vi "SMSMagnet.ProcEvents.vi"(0 "i ref in":refnum<vi>, 5 "error in (no error)":errorcluster) -> (14 "i ref out":refnum<vi>, 19 "error out":errorcluster)   [LabVIEW 2014, in "SMSMagnet.lvlib"]
doc: "This method is used to define the events the object will listen to. Add your own events here."
uses:
  SMSMagnet.lvlib
  CSCore/BaseProcess/BaseProcess.event definition.ctl
  CSCore/CAEObj/CAEObj.event definition.ctl
  CSCore/BaseProcess/BaseProcess.descriptor string definition.ctl
  CSCore/BaseProcess/BaseProcess.lvlib
  CSCore/CAEObj/CAEObj.lvlib
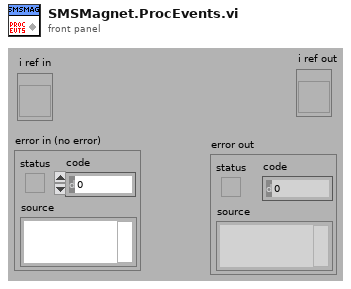
[diagram p1: front panel]
types:
  T1 = typedef "BaseProcess.lvlib/BaseProcess.event definition.ctl" = cluster{"CAEEvtDef":T2, "Data Descriptor":T3}
  T2 = typedef "CAEObj.lvlib/CAEObj.event definition.ctl" = cluster{"URL":string, "enable":bool, "ignoreResID":bool}
  T3 = typedef "BaseProcess.lvlib/BaseProcess.descriptor string definition.ctl" = string
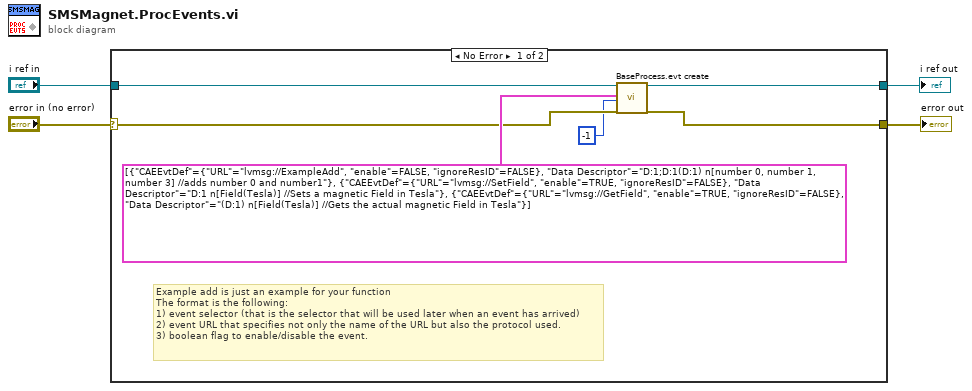
[diagram p0: block diagram]
diagram:
  n1 = case shown="No Error" "error in (no error)" {
    selector: "error in (no error)" -> [w6 w11]
    tunnel: "i ref in" -> [w10 w12]
    tunnel: [w9 w12] -> w3
    tunnel: [w8 w11] -> w2
    frame No Error {
      # "Example add is just an example for your function\nThe format is the following:\n1) event selector (that is the selector that will be used later when an event has arrived)\n2) event URL that specifies not only the name of the URL but also the protocol used.\n3) boolean flag to enable/disable the event."
      n2 = call "BaseProcess.evt create.vi"("i ref in"=w10, "newEvents"=T1[] [{"CAEEvtDef"={"URL"="lvmsg://ExampleAdd", "enable"=FALSE, "ignoreResID"=FALSE}, "Data Descriptor"="D:1;D:1(D:1) n[number 0, number 1, number 3] //adds number 0 and number1"}, {"CAEEvtDef"={"URL"="lvmsg://SetField", "enable"=TRUE, "ignoreResID"=FALSE}, "Data Descriptor"="D:1 n[Field(Tesla)] //Sets a magnetic Field in Tesla"}, {"CAEEvtDef"={"URL"="lvmsg://GetField", "enable"=TRUE, "ignoreResID"=FALSE}, "Data Descriptor"="(D:1) n[Field(Tesla)] //Gets the actual magnetic Field in Tesla"}] ("new events"), "ms timeout (10000)"=-1, "error in (no error)"=w6) -> ("i ref out"=w9:refnum<vi>, "error out"=w8:errorcluster)  [unwired: 12 in, 2 out]
    }
    frame Error {
    }
  }
  "i ref out" <- w3
  "error out" <- w2
